vi "getTopRectangle.vi"(0 "reference":refnum<class "ImplicitParameterNode.lvclass">, 5 "error in (no error)":errorcluster) -> (14 "reference out":refnum<class "ImplicitParameterNode.lvclass">, 15 "bounds":T1 {"height" format="%.2f"; "width" format="%.2f"; "y" format="%.2f"; "x" format="%.2f"}, 19 "error out":errorcluster)   [LabVIEW 2012, in "ImplicitParameterNode.lvclass"]
doc: "public Rectangle2D getTopRectangle()"
uses:
  <resource>/Framework/Providers/Open_GDS/UML/ImplicitParameterNode_class/ImplicitParameterNode.lvclass
  <resource>/Framework/Providers/Open_GDS/UML/General/Rectangle/Rectangle Rectangle2D.ctl
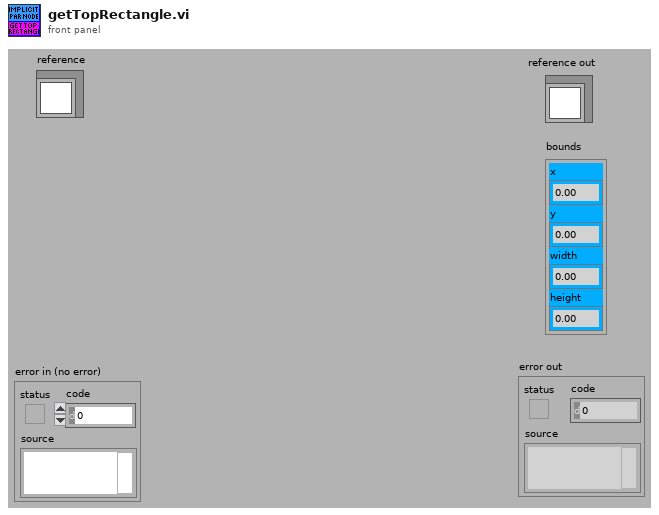
[diagram p1: front panel]
types:
  T1 = typedef "Rectangle Rectangle2D.ctl" = cluster{"x":dbl, "y":dbl, "width":dbl, "height":dbl}
  T2 = typedef "ImplicitParameterNode.lvclass/ObjectAttributes.ctl" = cluster{"Base class":T3, "topHeight":dbl, "name":refnum<class "MultiLineString.lvclass">, "DEFAULT_TOP_HEIGHT":i32, "DEFAULT_WIDTH":i32, "DEFAULT_HEIGHT":i32}
  T3 = typedef "RectangularNode.lvclass/ObjectAttributes.ctl" = cluster{"Base class":T4, "bounds":T1}
  T4 = typedef "AbstractNode.lvclass/ObjectAttributes.ctl" = cluster{"parent":refnum<class "AbstractNode.lvclass">, "children":refnum<class "AbstractNode.lvclass">[], "Hidden":bool}
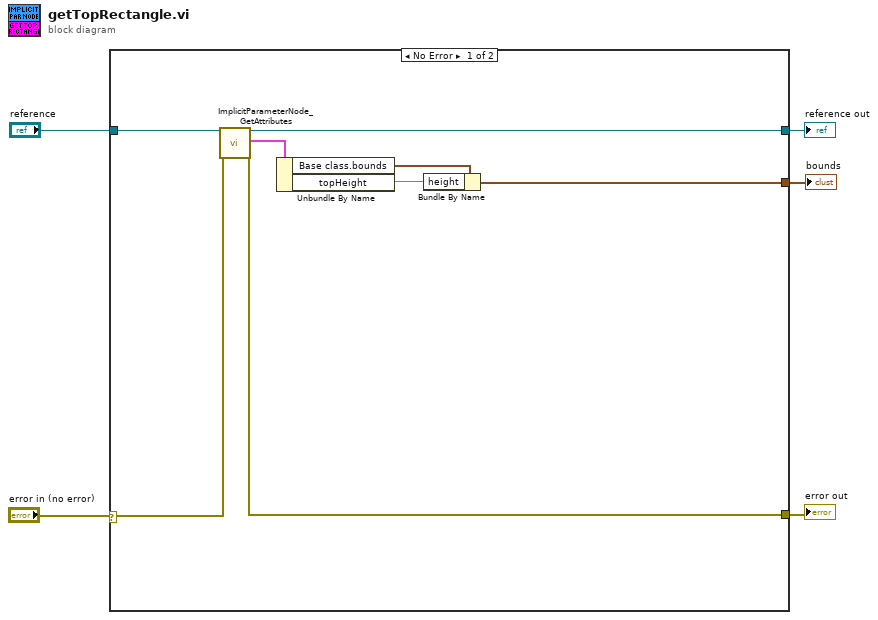
[diagram p0: block diagram]
diagram:
  n1 = case shown="No Error" "error in (no error)" {
    selector: "error in (no error)" -> [w10 w14]
    tunnel: "reference" -> [w13 w15]
    tunnel: [w12 w14] -> w4
    tunnel: [w11 w15] -> w3
    tunnel: [w9 _] -> w1
    frame No Error {
      n2 = call <resource>:"ImplicitParameterNode_GetAttributes.vi"("reference in"=w13, "error in (no error)"=w10) -> ("reference out"=w11:refnum<class "ImplicitParameterNode.lvclass">, "Attributes"=w8:T2, "error out"=w12:errorcluster)  [unwired: 15 out]
      n3 = Unbundle By Name(w8) -> ("Base class.bounds"=w7:T1, "topHeight"=w6:dbl)
      n4 = Bundle By Name(cluster=w7, "height"=w6) -> (w9:T1)
    }
    frame Error {
    }
  }
  "reference out" <- w3
  "error out" <- w4
  "bounds" <- w1
